vi "Create Transfer Group Configuration.vi"(6 "group timing (dec:1, off: 0)":T5={"priority"=0, "decimation"=1, "offset"=0}, 7 "base group name (group)":string="group", 9 "direction":T4, 10 "channel count per transfer":i32, 11 "transfer configs":T2(array[cluster])) -> (3 "Transfer Group":T3={"name"="", "direction"=enum."Tx", "cycle timing"={"priority"=0, "decimation"=1, "offset"=0}, "Transfers"=[], "settings"=[]})   [LabVIEW 2017]
uses:
  Built/Windows/Engine/DSF.Engine.lvlibp/DSF Configuration API/1.0.0/Public/Controls/DSF Timing Info.ctl
  Built/Windows/Engine/DSF.Engine.lvlibp/DSF Configuration API/1.0.0/Public/Controls/DSF Direction.ctl
  Built/Windows/Engine/DSF.Engine.lvlibp/DSF Configuration API/1.0.0/Public/Controls/DSF Engine Transfer Group Configuration.ctl
  Built/Windows/Engine/DSF.Engine.lvlibp/DSF Configuration API/1.0.0/Public/Controls/DSF Engine Transfer Configuration.ctl
  Built/Windows/Engine/DSF.Engine.lvlibp/DSF Configuration API/1.0.0/Public/Controls/DSF Byte Order.ctl
  Built/Windows/Engine/DSF.Engine.lvlibp/DSF Configuration API/1.0.0/Public/Controls/DSF Engine Channel Configuration.ctl
  Built/Windows/Engine/DSF.Engine.lvlibp/DSF Configuration API/1.0.0/Public/Controls/DSF Data Type.ctl
  Built/Windows/Engine/DSF.Engine.lvlibp/DSF Configuration API/1.0.0/Public/Controls/DSF Settings Info.ctl
  Built/Windows/Engine/DSF.Engine.lvlibp/DSF Configuration API/1.0.0/DSF Configuration API.lvlib
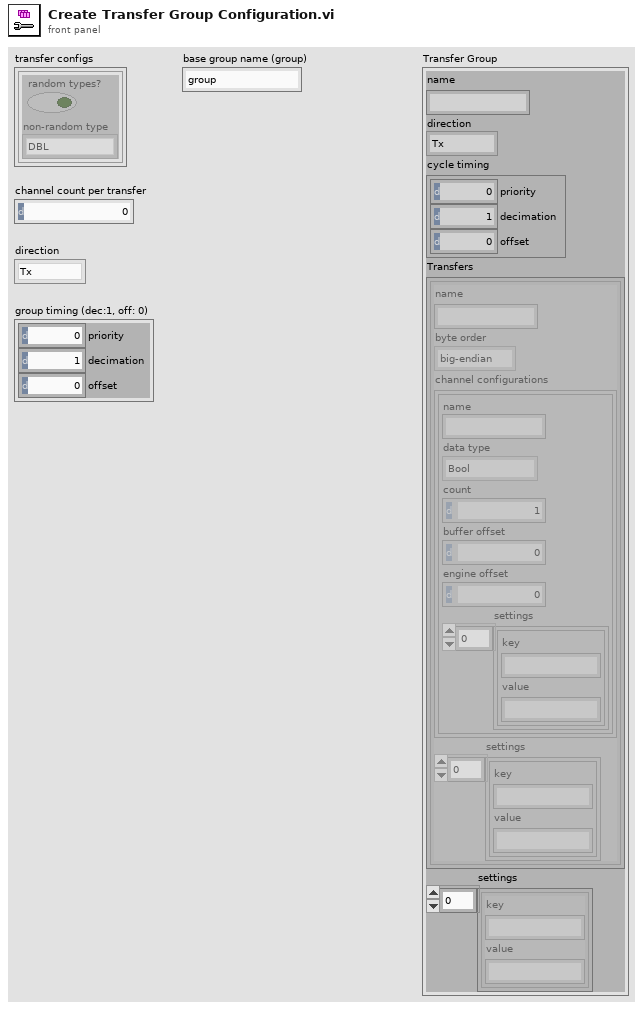
[diagram p1: front panel]
types:
  T1 = typedef "DSF.Engine.lvlibp/DSF Configuration API.lvlib/DSF Data Type.ctl" = enum8{"Bool", "SGL", "DBL", "I8", "I16", "I32", "I64", "U8", "U16", "U32", "U64"}
  T2 = cluster{"random types?":bool, "non-random type":T1}[]
  T3 = typedef "DSF.Engine.lvlibp/DSF Configuration API.lvlib/DSF Engine Transfer Group Configuration.ctl" = cluster{"name":string, "direction":T4, "cycle timing":T5, "Transfers":T6[], "settings":T9}
  T4 = typedef "DSF.Engine.lvlibp/DSF Configuration API.lvlib/DSF Direction.ctl" = enum8{"Tx", "Rx"}
  T5 = typedef "DSF.Engine.lvlibp/DSF Configuration API.lvlib/DSF Timing Info.ctl" = cluster{"priority":u64, "decimation":u64, "offset":u64}
  T6 = typedef "DSF.Engine.lvlibp/DSF Configuration API.lvlib/DSF Engine Transfer Configuration.ctl" = cluster{"name":string, "byte order":T7, "channel configurations":T8[], "settings":T9}
  T7 = typedef "DSF.Engine.lvlibp/DSF Configuration API.lvlib/DSF Byte Order.ctl" = enum8{"big-endian", "little-endian"}
  T8 = typedef "DSF.Engine.lvlibp/DSF Configuration API.lvlib/DSF Engine Channel Configuration.ctl" = cluster{"name":string, "data type":T1, "count":u64, "buffer offset":u64, "engine offset":u64, "settings":T9}
  T9 = typedef "DSF.Engine.lvlibp/DSF Configuration API.lvlib/DSF Settings Info.ctl" = cluster{"key":string, "value":string}[]
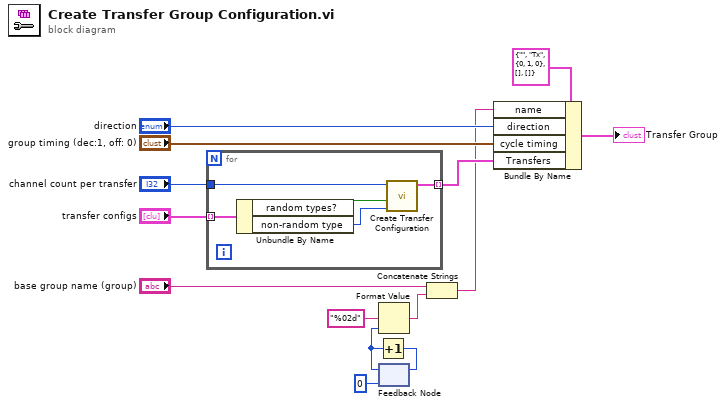
[diagram p0: block diagram]
diagram:
  n1 = for {
    tunnel: "channel count per transfer" -> [w19]
    tunnel: [w18] -> w2 mode=indexing
    tunnel: "transfer configs" -> [w17] mode=indexing
    n2 = Unbundle By Name(w17) -> ("random types?"=w16:bool, "non-random type"=w15:T1)
    n3 = call "Create Transfer Configuration.vi"("non-random type (DBL)"=w15, "random types? (F)"=w16, "channel count per transfer"=w19) -> ("Transfers"=w18:T6)  [unwired: 8 in]
  }
  n4 = feedback #1(0) -> (w13:i32)
  n5 = Increment(x=w13) -> (x+1=w11:i32)
  n6 = Format Value(format string="%02d", value (0)=w13) -> (output string=w7:string)  [unwired: 1 in]
  n7 = feedback-in #1(w11) -> ()
  n8 = Concatenate Strings("base group name (group)", w7) -> (w1:string)
  n9 = Bundle By Name(cluster=T3 {"name"="", "direction"=enum."Tx", "cycle timing"={"priority"=0, "decimation"=1, "offset"=0}, "Transfers"=[], "settings"=[]} ("Transfer Groups"), "name"=w1, "direction"="direction", "cycle timing"="group timing (dec:1, off: 0)", "Transfers"=w2) -> (→"Transfer Group":T3)
